vi "size.vi"(8 "Error In":errorcluster, 11 "QPixmap In":refnum<class "QPixmap.lvclass">) -> (0 "Error Out":errorcluster, 2 "Value":T1, 3 "QPixmap Out":refnum<class "QPixmap.lvclass">)   [LabVIEW 2014, in "QPixmap.lvclass"]
doc: "LabVIEW-specific documentation is not yet available. See <b>http://doc.qt.io/qt-5/QPixmap.html#size</b>"
uses:
  QPixmap.lvclass
  LQ Core/QSize.ctl
  LQ Core/LQSerialData/LQSerialData.lvclass/LQSerialData.ctl
  LQ Core/LQ Core.lvlib
  LQ Core/LQSerialData/LQSerialData.lvclass
panel:
  # "Copyright (c) 2016 Sze Howe Koh\n\nThis Source Code Form is subject to the terms of the Mozilla Public\nLicense, v. 2.0. If a copy of the MPL was not distributed with this\nfile, You can obtain one at http://mozilla.org/MPL/2.0/."
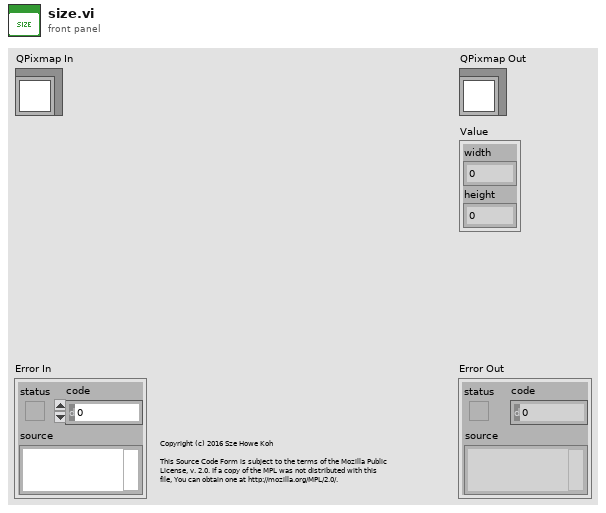
[diagram p1: front panel]
types:
  T1 = typedef "QSize.ctl" = cluster{"width":i32, "height":i32}
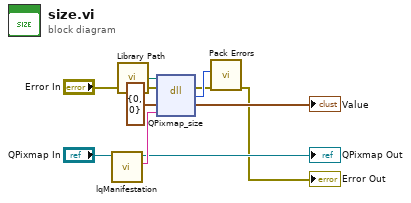
[diagram p0: block diagram]
diagram:
  n1 = call "lqManifestation.vi"("LQSerialData in"="QPixmap In") -> ("Manifestation"=w7:string, "LQSerialData out"=→"QPixmap Out":refnum<class "QPixmap.lvclass">)  [unwired: 9 in]
  n2 = call "Library Path.vi"() -> ("Library Path"=w4:path)
  n3 = dll-call lib="?" fn="QPixmap_size"(path in=w4, error in="Error In", "_retVal"=T1 {"width"=0, "height"=0} ("retVal"), "_instance"=w7) -> (error out=w2:errorcluster, w3:i32, "_retVal"=→"Value":T1)  [unwired: 2 in, 1 out]
  n4 = call "Pack Errors.vi"("Error In"=w2, "Error Code"=w3) -> ("Error Out"=→"Error Out":errorcluster)  [unwired: 9 in]
